vi "setVoltageOff.vi"(9 "Mode":bool, 10 "Current Temperature (simulated)":refnum<vi>, 11 "Room Temperature (K)":refnum<vi>) -> (3 "Voltage":dbl)   [LabVIEW 2013]
uses:
  Controls/FGV Function.ctl
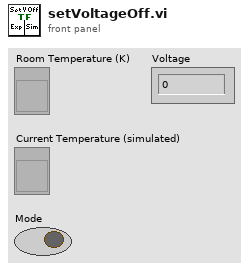
[diagram p1: front panel]
types:
  T1 = typedef "FGV Function.ctl" = enum16{"Initiate", "Read", "Set On", "Set Off"}
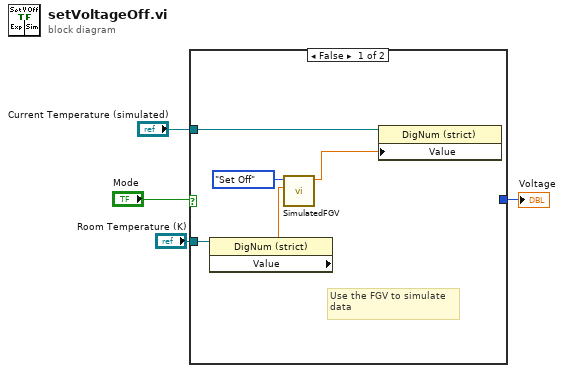
[diagram p0: block diagram]
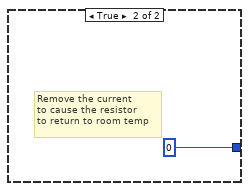
[diagram p2: hidden frame]
diagram:
  n1 = case shown="False" "Mode" {
    tunnel: [_ 0] -> w4
    tunnel: "Room Temperature (K)" -> [w6 _]
    tunnel: "Current Temperature (simulated)" -> [w5 _]
    frame False {
      # "Use the FGV to simulate \ndata"
      n2 = property on="Property Node" class="DigNum (strict)"(reference=w6) -> ("Value"=w9:dbl)  [unwired: 1 in, 2 out]
      n3 = call "SimulatedFGV.vi"("Starting Temperature"=w9, "FGV Function"=FGV_Function."Set Off") -> ("Current Temperature"=w7:dbl)  [unwired: 9 in]
      n4 = property on="Property Node" class="DigNum (strict)"(reference=w5, "Value"=w7) -> ()  [unwired: 1 in, 2 out]
    }
    frame True {
      # "Remove the current\nto cause the resistor\nto return to room temp"
    }
  }
  "Voltage" <- w4
